vi "Check Master and Slave Health.vi"(6 "Timeout duration":dbl, 8 "Error In":errorcluster, 9 "Master and Slave VI names":T1, 10 "Slave timer names array":string[](array[string]), 11 "Master timer names array":string[](array[string])) -> (0 "Error Out":errorcluster, 1 "Unresponsive Slaves":string[](array[string]), 2 "Unresponsive Masters":string[](array[string]), 3 "Any Master or Slave Unresponsive?":bool)   [LabVIEW 2012]
doc: "SciScan 1.2 160622\nThis VI checks if any of the ENABLED timers have timed out.\nIn the event for a timeout, a Boolean is set, and the type of timeout (VI state) is output.\n\nNotes:\n-------s\n1. This VI is customised to work with the Macro module of SciScan as it checks specifically for timers related to this module (eg. <VI name + _listen_for_MASTER_HB>)\n2. For this VI to work, the timer must be initialized (Once in the main aplication), and the countdown time set to the desired value before running this VI"
uses:
  CommonResource VIs/Timing/Timer Commands.ctl
  SubVIs/Broken Chain FGV Command.ctl
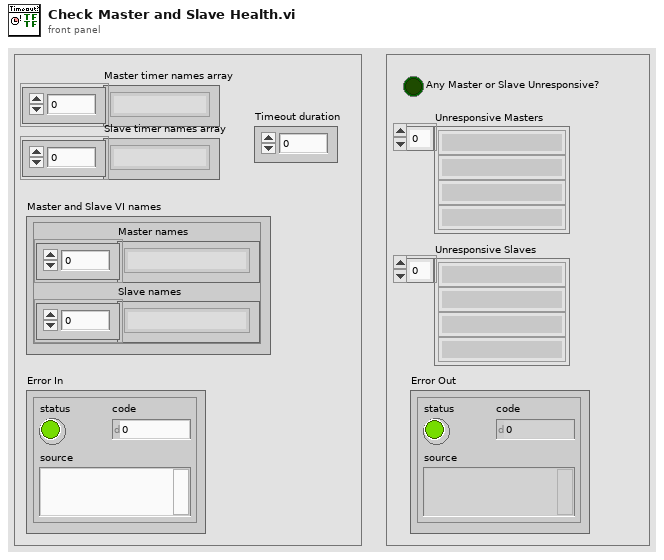
[diagram p1: front panel]
types:
  T1 = cluster{"Master names":string[], "Slave names":string[]}
  T2 = typedef "Broken Chain FGV Command.ctl" = enum16{"Initialize", "Update VI status", "Get All VI status"}
  T3 = typedef "Timer Commands.ctl" = enum16{"Clear All", "Start", "Pause", "Check Time"}
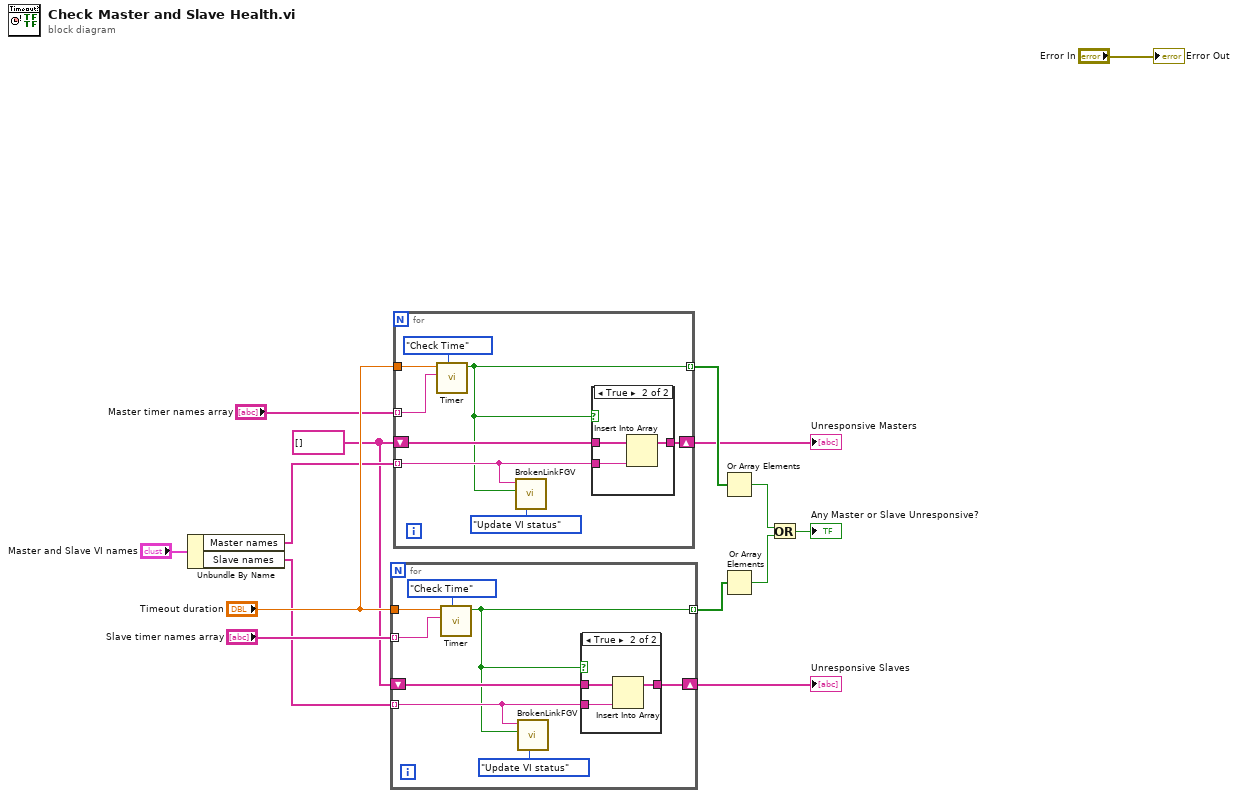
[diagram p0: block diagram]
diagram:
  w3 = string[] [] ("Master names")
  n1 = Unbundle By Name("Master and Slave VI names") -> ("Master names"=w5:string[], "Slave names"=w4:string[])
  n2 = for {
    tunnel: "Timeout duration" -> [w22]
    tunnel: [w16] -> w7 mode=indexing
    tunnel: "Slave timer names array" -> [w21] mode=indexing
    tunnel: w4 -> [w17] mode=indexing
    shift-right: [w19] -> w2
    shift-left: w3 -> [w20]
    n3 = call "Timer.vi"("Timer Command"=Timer_Commands."Check Time", "VI name (Optional)"=w21, "Set Time IN (s)"=w22) -> ("Complete?"=w16:bool)  [unwired: 3 in, 5 out]
    n4 = call "BrokenLinkFGV.vi"("Broken Chain FGV Action"=Broken_Chain_FGV_Command."Update VI status", "Broken?"=w16, "String"=w17) -> ()  [unwired: 6 in, 3 out]
    n5 = case shown="True" w16 {
      tunnel: w20 -> [w24 w27]
      tunnel: [w24 w26] -> w19
      tunnel: w17 -> [_ w25]
      frame False {
      }
      frame True {
        n6 = Insert Into Array(array=w27, new element=w25) -> (w26:string[])  [unwired: 1 in]
      }
    }
  }
  "Unresponsive Slaves" <- w2
  n7 = for {
    tunnel: [w29] -> w13 mode=indexing
    tunnel: "Timeout duration" -> [w34]
    tunnel: "Master timer names array" -> [w33] mode=indexing
    tunnel: w5 -> [w30] mode=indexing
    shift-right: [w31] -> w1
    shift-left: w3 -> [w32]
    n8 = call "Timer.vi"("Timer Command"=Timer_Commands."Check Time", "VI name (Optional)"=w33, "Set Time IN (s)"=w34) -> ("Complete?"=w29:bool)  [unwired: 3 in, 5 out]
    n9 = call "BrokenLinkFGV.vi"("Broken Chain FGV Action"=Broken_Chain_FGV_Command."Update VI status", "Broken?"=w29, "String"=w30) -> ()  [unwired: 6 in, 3 out]
    n10 = case shown="True" w29 {
      tunnel: w32 -> [w36 w39]
      tunnel: [w36 w38] -> w31
      tunnel: w30 -> [_ w37]
      frame False {
      }
      frame True {
        n11 = Insert Into Array(array=w39, new element=w37) -> (w38:string[])  [unwired: 1 in]
      }
    }
  }
  "Unresponsive Masters" <- w1
  n12 = Or Array Elements(Boolean array=w13) -> (logical OR=w10:bool)
  n13 = Or Array Elements(Boolean array=w7) -> (logical OR=w9:bool)
  n14 = Or(x=w10, y=w9) -> (x .or. y?=→"Any Master or Slave Unresponsive?":bool)
  "Error Out" <- "Error In"
